vi "Secret_Code.vi"() -> ()   [LabVIEW 2014]
uses:
  <vilib>/event_ctls.llb/lveventtype.ctl
panel:
  out "cluster":T1
  out "initialized array":bool[](array[boolean])
  out "ScanCode":i16
  in  "stop":bool
  out "Numeric":i32
  out "JMS":bool
  out "Char":i16
  out "S#":i16
  out "S":bool
  out "M#":i16
  out "M":bool
  out "J #":i16
  out "J":bool
  out "x .and. y?":bool
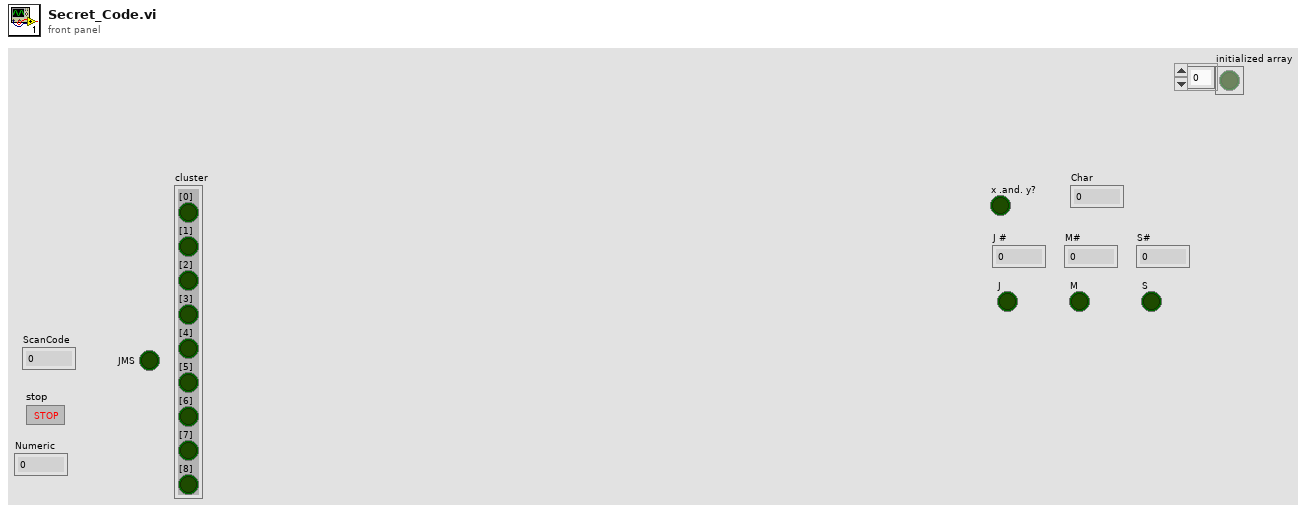
[diagram p1: front panel]
types:
  T1 = cluster{"[0]":bool, "[1]":bool, "[2]":bool, "[3]":bool, "[4]":bool, "[5]":bool, "[6]":bool, "[7]":bool, "[8]":bool}
  T2 = cluster{"Shift":bool, "Ctrl":bool, "Alt":bool, "Cmd":bool, "Opt":bool}
  T3 = typedef "lveventtype.ctl" = enum32{"Null", "Timeout", "Annotation Menu Selection", "Annotation Menu Selection?", "App Instance Close", "App Instance Close?", "Autoscale Range Change", "Bookmark Info Change", "Cell Edit", "Cell Edit?", "Cursor Grab", "Cursor Grab?", "Cursor Menu Selection", "Cursor Menu Selection?", "Cursor Move", "Cursor Release", "Data Change", "Direction Change", "Display State Change", "Drag Ended", "Drag Enter", "Drag Leave", "Drag Over", "Drag Source Update", "Drag Starting", "Drag Starting?", "Drop", "Exec State Change", "Key Down", "Key Down?", "Key Repeat", "Key Repeat?", "Key Up", "Listbox Double Click", "Menu Activation?", "Menu Selection (App)", "Menu Selection? (App)", "Menu Selection (User)", "Mouse Down", "Mouse Down?", "Mouse Enter", "Mouse Leave", "Mouse Move", "Mouse Up", "Mouse Wheel", "NI Security User Change (App)", "Pane Size", "Panel Close", "Panel Close?", "Panel Resize", "Plot Attribute Change", "Scale Range Change", "Shortcut Menu Activation?", "Shortcut Menu Selection (App)", "Shortcut Menu Selection? (App)", "Shortcut Menu Selection (User)", "Tree Double Click", "Tree Drag", "Tree Drag?", "Tree Drop", "Tree Drop?", "Tree Item Close", "Tree Item Close?", "Tree Item Open", "Tree Item Open?", "User Event", "Value Change"}
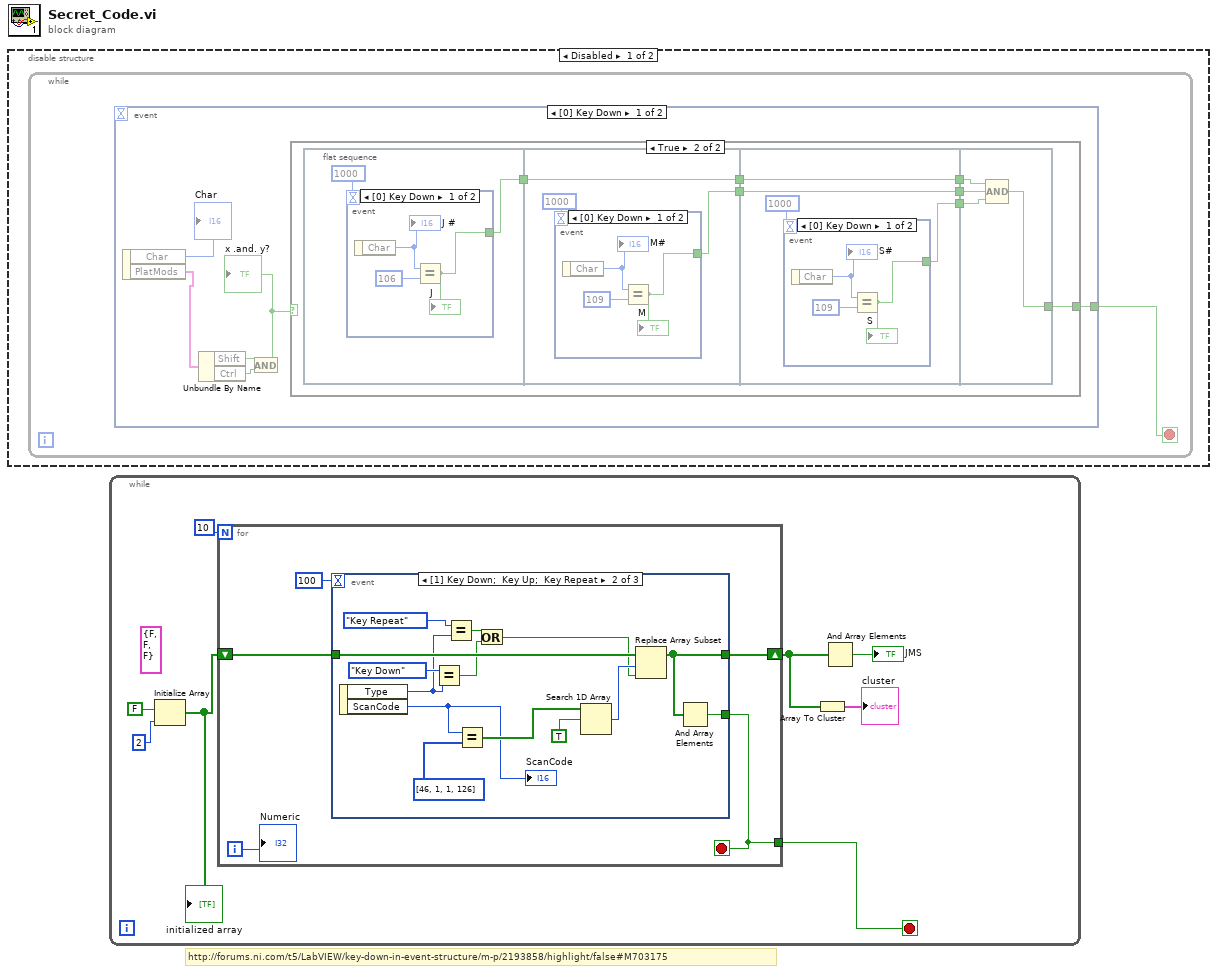
[diagram p0: block diagram]
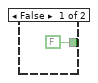
[diagram p2: hidden frame]
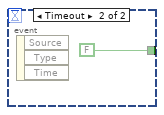
[diagram p3: hidden frame]
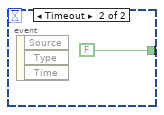
[diagram p4: hidden frame]
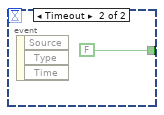
[diagram p5: hidden frame]
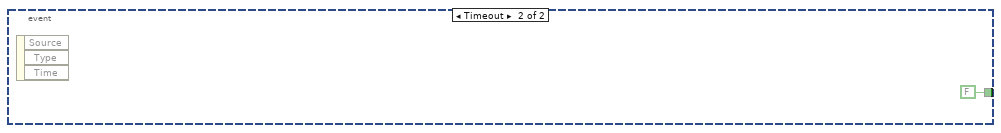
[diagram p6: hidden frame]
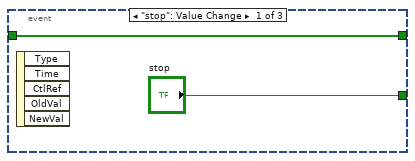
[diagram p8: hidden frame]
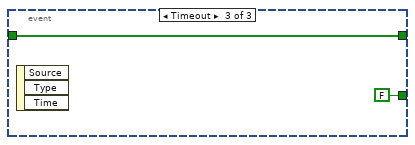
[diagram p9: hidden frame]
diagram:
  # "http://forums.ni.com/t5/LabVIEW/key-down-in-event-structure/m-p/2193858/highlight/false#M703175"
  n1 = disable-structure shown="Disabled" {
    frame Disabled {
      n2 = while {
        stop <- w1 stop-if-true
        n3 = event shown="[0] Key Down" {
          selector: _ -> [_ _]
          dyn-events: _ -> [_ _]
          timeout: _ -> [_ _]
          tunnel: [w3 FALSE] -> w1
          event Key Down {
            n4 = event-data() -> ("Char"=→"Char":i16, "PlatMods"=w7:T2)  [unwired: 1 in]
            n5 = Unbundle By Name(w7) -> ("Shift"=w6:bool, "Ctrl"=w5:bool)
            n6 = And(x=w6, y=w5) -> (x .and. y?=w4:bool)
            "x .and. y?" <- w4
            n7 = case shown="True" w4 {
              tunnel: [FALSE w9] -> w3
              frame False {
              }
              frame True {
                n8 = flat-sequence {
                  tunnel: [w16] -> w15
                  tunnel: [w24] -> w14
                  tunnel: w15 -> [w24]
                  tunnel: [w22] -> w13
                  tunnel: [w32] -> w12
                  tunnel: w14 -> [w32]
                  tunnel: [w31] -> w11
                  tunnel: w13 -> [w31]
                  tunnel: [w29] -> w10
                  tunnel: w12 -> [w40]
                  tunnel: w11 -> [w39]
                  tunnel: w10 -> [w38]
                  tunnel: [w37] -> w9
                  frame #0 {
                    n9 = event shown="[0] Key Down" {
                      selector: _ -> [_ _]
                      dyn-events: _ -> [_ _]
                      timeout: 1000 -> [_ _]
                      tunnel: [w18 FALSE] -> w16
                      event Key Down {
                        n10 = event-data() -> ("Char"=w19:i16)  [unwired: 1 in]
                        "J #" <- w19
                        n11 = Equal?(x=w19, y=i16 106) -> (x = y?=w18:bool)
                        "J" <- w18
                      }
                      event Timeout {
                        n12 = event-data() -> ()  [unwired: 1 in, 3 out]
                      }
                    }
                  }
                  frame #1 {
                    n13 = event shown="[0] Key Down" {
                      selector: _ -> [_ _]
                      dyn-events: _ -> [_ _]
                      timeout: 1000 -> [_ _]
                      tunnel: [w25 FALSE] -> w22
                      event Key Down {
                        n14 = event-data() -> ("Char"=w26:i16)  [unwired: 1 in]
                        "M#" <- w26
                        n15 = Equal?(x=w26, y=i16 109) -> (x = y?=w25:bool)
                        "M" <- w25
                      }
                      event Timeout {
                        n16 = event-data() -> ()  [unwired: 1 in, 3 out]
                      }
                    }
                  }
                  frame #2 {
                    n17 = event shown="[0] Key Down" {
                      selector: _ -> [_ _]
                      dyn-events: _ -> [_ _]
                      timeout: 1000 -> [_ _]
                      tunnel: [w33 FALSE] -> w29
                      event Key Down {
                        n18 = event-data() -> ("Char"=w34:i16)  [unwired: 1 in]
                        "S#" <- w34
                        n19 = Equal?(x=w34, y=i16 109) -> (x = y?=w33:bool)
                        "S" <- w33
                      }
                      event Timeout {
                        n20 = event-data() -> ()  [unwired: 1 in, 3 out]
                      }
                    }
                  }
                  frame #3 {
                    n21 = Compound Arithmetic op=AND(w40, w39, w38) -> (w37:bool)
                  }
                }
              }
            }
          }
          event Timeout {
            n22 = event-data() -> ()  [unwired: 1 in, 3 out]
          }
        }
      }
    }
    frame Enabled {
    }
  }
  n23 = while {
    stop <- w48 stop-if-true
    (unwired) cluster{"[0]":bool, "[1]":bool, "[2]":bool} {"[0]"=FALSE, "[1]"=FALSE, "[2]"=FALSE} ("cluster")
    n24 = Initialize Array(FALSE ("[2]"), 2 ("dimension size")) -> (w44:bool[])
    "initialized array" <- w44
    n25 = for {
      N: 10 -> [_]
      tunnel: [w52] -> w48
      shift-right: [w54] -> w43
      shift-left: w44 -> [w53]
      i -> [w51]
      stop <- w52 stop-if-true
      n26 = event shown="[1] Key Down;  Key Up;  Key Repeat" {
        selector: _ -> [_ _ _]
        dyn-events: _ -> [_ _ _]
        timeout: 100 -> [_ _ _]
        tunnel: ["stop" w57 FALSE ("stop")] -> w52
        tunnel: [w55 w58 w72] -> w54
        tunnel: w53 -> [w55 w64 w72]
        event "stop": Value Change {
          n27 = event-data() -> ()  [unwired: 1 in, 5 out]
        }
        event Key Down; Key Up; Key Repeat {
          n28 = event-data() -> ("Type"=w59:T3, "ScanCode"=w65:i16)  [unwired: 1 in]
          "ScanCode" <- w65
          n29 = Equal?(x=lveventtype."Key Down" ("Type"), y=w59) -> (x = y?=w63:bool)
          n30 = Equal?(x=lveventtype."Key Repeat" ("Type"), y=w59) -> (x = y?=w61:bool)
          n31 = Equal?(x=w65, y=i16[] [46, 1, 1, 126]) -> (x = y?=w68:bool[])
          n32 = Or(x=w61, y=w63) -> (x .or. y?=w62:bool)
          n33 = Search 1D Array(1D array=w68, element=TRUE) -> (index of element=w66:i32)  [unwired: 1 in]
          n34 = Replace Array Subset(array=w64, new element=w62, index=w66) -> (w58:bool[])
          n35 = And Array Elements(Boolean array=w58) -> (logical AND=w57:bool)
        }
        event Timeout {
          n36 = event-data() -> ()  [unwired: 1 in, 3 out]
        }
      }
      "Numeric" <- w51
    }
    n37 = Array To Cluster(array=w43) -> (cluster=→"cluster":T1)
    n38 = And Array Elements(Boolean array=w43) -> (logical AND=→"JMS":bool)
  }
